vi "PhotonCamera_GetLatestResult.vi"(11 "CameraName":string) -> (1 "HasTargets":bool, 3 "PipelineResult":T1 {"Targets"."AltCameraToTarget"."ROTATION"."SIN" format="%13.4f"; "Targets"."AltCameraToTarget"."ROTATION"."COS" format="%13.4f"; "Targets"."AltCameraToTarget"."ROTATION"."VALUE" format="%13.4f"; "Targets"."AltCameraToTarget"."TRANSLATION"."Y" format="%14.3f"; "Targets"."AltCameraToTarget"."TRANSLATION"."X" format="%14.3f"; "Targets"."BestCameraToTarget"."ROTATION"."SIN" format="%13.4f"; "Targets"."BestCameraToTarget"."ROTATION"."COS" format="%13.4f"; "Targets"."BestCameraToTarget"."ROTATION"."VALUE" format="%13.4f"; "Targets"."BestCameraToTarget"."TRANSLATION"."Y" format="%14.3f"; "Targets"."BestCameraToTarget"."TRANSLATION"."X" format="%14.3f"})   [LabVIEW 2020, in "PhotonVisionLib.lvlib"]
doc: "Returns the latest pipeline result.\n\nInputs:\n - cameraName -- The nickname of the camera (found in the PhotonVision UI).\n\nOutputs:\n - PipelineResult -- The latest pipeline result data cluster\n - HasTargets -- Boolean indicating if any targets were found"
uses:
  PhotonVisionLib.lvlib
  <vilib>/Rock Robotics/Network Tables/NT Read Raw.vi
  TypeDef/PhotonPipelineResultType.ctl
  TypeDef/PhotonTrackedTargetType.ctl
  TypeDef/TargetCornerType.ctl
  <vilib>/Rock Robotics/WPI/ThirdParty/JAS_Junk/TrajLib/TypeDef/TRANSFORM2D.ctl
  <vilib>/Rock Robotics/WPI/ThirdParty/JAS_Junk/TrajLib/TypeDef/TRANSLATION2D.ctl
  <vilib>/Rock Robotics/WPI/ThirdParty/JAS_Junk/TrajLib/TypeDef/ROTATION2D.ctl
  <vilib>/Rock Robotics/WPI/ThirdParty/JAS_Junk/TrajLib/Trajectory_Library.lvlib
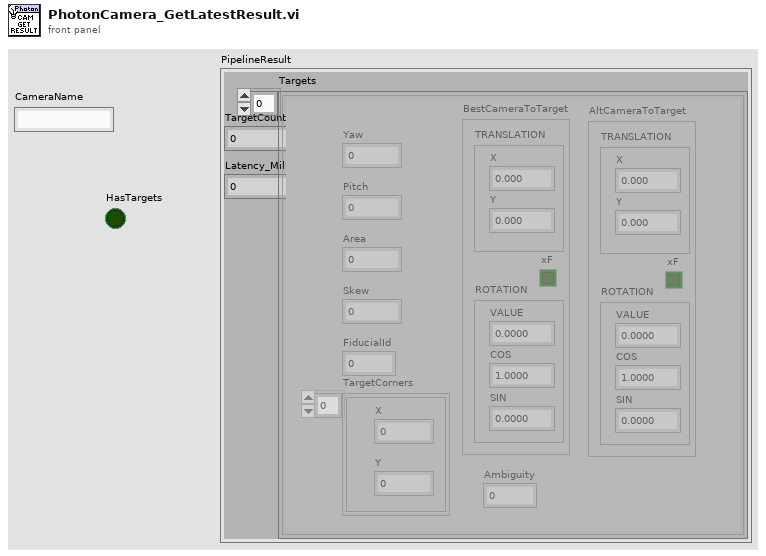
[diagram p1: front panel]
types:
  T1 = typedef "PhotonVisionLib.lvlib/PhotonPipelineResultType.ctl" = cluster{"TargetCount":i32, "Latency_MilliSec":dbl, "Targets":T2[]}
  T2 = typedef "PhotonVisionLib.lvlib/PhotonTrackedTargetType.ctl" = cluster{"Yaw":dbl, "Pitch":dbl, "Area":dbl, "Skew":dbl, "TargetCorners":T3[], "BestCameraToTarget":T4, "FiducialId":i32, "AltCameraToTarget":T4, "Ambiguity":dbl}
  T3 = typedef "PhotonVisionLib.lvlib/TargetCornerType.ctl" = cluster{"X":dbl, "Y":dbl}
  T4 = typedef "Trajectory_Library.lvlib/TRANSFORM2D.ctl" = cluster{"TRANSLATION":T5, "ROTATION":T6, "xF":bool}
  T5 = typedef "Trajectory_Library.lvlib/TRANSLATION2D.ctl" = cluster{"X":dbl, "Y":dbl}
  T6 = typedef "Trajectory_Library.lvlib/ROTATION2D.ctl" = cluster{"VALUE":dbl, "COS":dbl, "SIN":dbl}
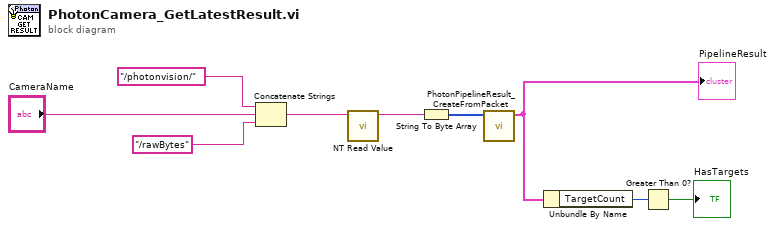
[diagram p0: block diagram]
diagram:
  n1 = Concatenate Strings("/photonvision/", "CameraName", "/rawBytes") -> (w6:string)
  n2 = call-poly <vilib>:"NT Read Value.vi"("Name"=w6) -> ("Raw"=w5:string)  [unwired: 9 in, 1 out]
  n3 = String To Byte Array(string=w5) -> (unsigned byte array=w4:u8[])
  n4 = call "PhotonPipelineResult_CreateFromPacket.vi"("RawData"=w4) -> ("PhotonPipelineResult"=w3:T1)  [unwired: 10 in]
  "PipelineResult" <- w3
  n5 = Unbundle By Name(w3) -> ("TargetCount"=w2:i32)
  n6 = Greater Than 0?(x=w2) -> (x > 0?=→"HasTargets":bool)
